vi "richards_fast_tracking_find_dll.vi"() -> (3 "appended path":path)   [LabVIEW 2010]
doc: "This VI locates the DLL for symmetry transforms (either in the same directory, the directory above or the system directory)."
uses:
  <vilib>/Utility/sysdir.llb/System Directory Type.ctl
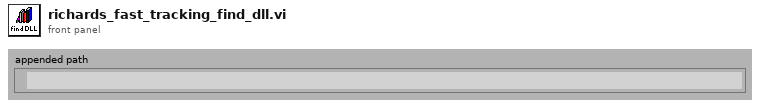
[diagram p1: front panel]
types:
  T1 = typedef "System Directory Type.ctl" = i32
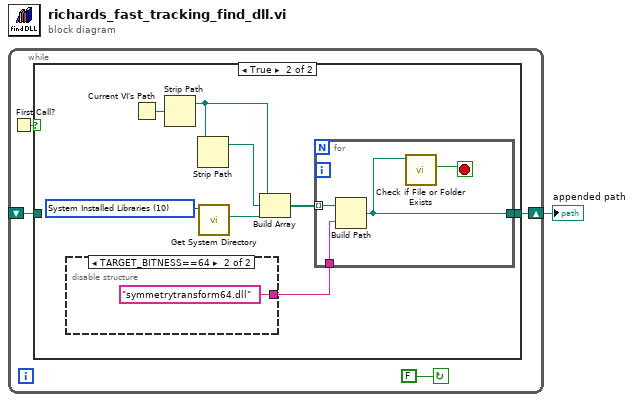
[diagram p0: block diagram]
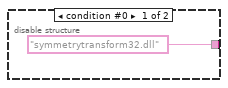
[diagram p3: hidden frame]
diagram:
  n1 = while {
    shift-right: [w3] -> w1
    shift-left: _ -> [w2]
    stop <- FALSE continue-if-true
    n2 = First Call?() -> (First Call?: T/F=w4:bool)
    n3 = case shown="True" w4 {
      tunnel: [w6 w8] -> w3
      tunnel: w2 -> [w6 _]
      frame False {
      }
      frame True {
        w14 = T1 10 items=["User Home"=0, "User Desktop"=1, "User Documents"=2, "User Application Data"=3, "User Preferences"=4, "User Temporary"=5, "Public Documents"=6, "Public Application Data"=7, "Public Preferences"=8, "Public Cache"=13, "System Core Libraries"=9, "System Installed Libraries"=10, "Application Files"=11, "Boot Volume Root"=12] ("system directory type")
        n4 = disable-structure shown="TARGET_BITNESS==64" {
          disable-tunnel: ["symmetrytransform32.dll" ("name or relative path") "symmetrytransform64.dll" ("name or relative path")] -> w7
          frame condition #0 {
          }
          frame condition #1 (active) {
          }
        }
        n5 = Current VI's Path() -> (path=w13:path)
        n6 = Strip Path(path=w13) -> (stripped path=w10:path)  [unwired: 1 out]
        n7 = Strip Path(path=w10) -> (stripped path=w11:path)  [unwired: 1 out]
        n8 = call <vilib>:"Get System Directory.vi"("system directory type"=w14) -> ("system directory"=w12:path)  [unwired: 10 in]
        n9 = Build Array(w10, w11, w12) -> (w9:path[])
        n10 = for {
          tunnel: w9 -> [w20] mode=indexing
          tunnel: [w18] -> w8
          tunnel: w7 -> [w17]
          stop <- w19 stop-if-true
          n11 = Build Path(base path=w20, name or relative path=w17) -> (appended path=w18:path)
          n12 = call <vilib>:"Check if File or Folder Exists.vi"("path"=w18) -> ("file or folder exists?"=w19:bool)  [unwired: 8 in, 2 out]
        }
      }
    }
  }
  "appended path" <- w1
